vi "Init Prefs.vi"(8 "error in (no error)":errorcluster, 11 "SB App in":refnum<class "SB App.lvclass">) -> (0 "error out":errorcluster, 3 "SB App out":refnum<class "SB App.lvclass">)   [LabVIEW 2020, in "SB App.lvlib" / "SB App.lvclass"]
uses:
  SB App.lvclass
  SB App.lvclass/SB App.ctl
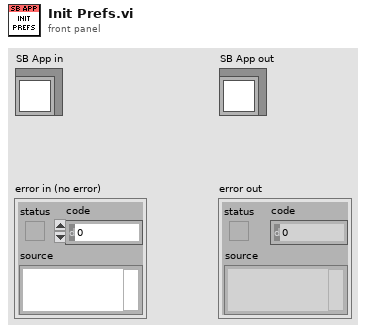
[diagram p1: front panel]
types:
  T1 = enum16{"open", "replace", "create", "open or create", "replace or create", "replace or create with confirmation"}
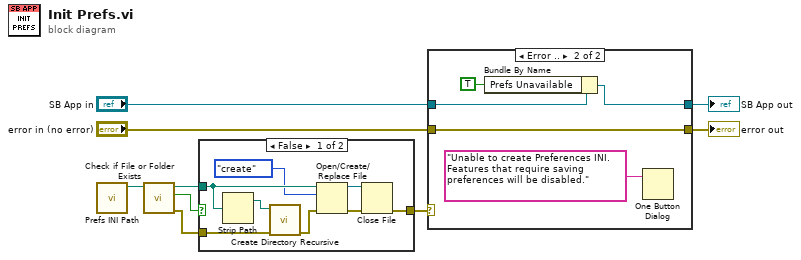
[diagram p0: block diagram]
diagram:
  n1 = call "Prefs INI Path.vi"() -> ("Prefs INI"=w9:path)  [unwired: 11 in]
  n2 = call <vilib>:"Check if File or Folder Exists.vi"("path"=w9) -> ("error out"=w6:errorcluster, "file or folder exists?"=w8:bool, "dup path"=w7:path)  [unwired: 8 in]
  n3 = case shown="False" w8 {
    tunnel: w7 -> [w15 _]
    tunnel: w6 -> [w17 w18]
    tunnel: [w10 w18] -> w5
    frame False {
      n4 = Strip Path(path=w15) -> (stripped path=w16:path)  [unwired: 1 out]
      n5 = call <vilib>:"Create Directory Recursive.vi"("error in (no error)"=w17, "directory"=w16) -> ("error out"=w14:errorcluster)  [unwired: 3 in, 2 out]
      n6 = Open/Create/Replace File(file path (use dialog)=w15, error in=w14, operation (0:open)=T1."create") -> (refnum out=w11:refnum<file>, error out=w12:errorcluster)  [unwired: 3 in, 1 out]
      n7 = Close File(refnum=w11, error in=w12) -> (error out=w10:errorcluster)  [unwired: 1 out]
    }
    frame True {
    }
  }
  n8 = case shown="Error .." w5 {
    tunnel: "error in (no error)" -> [w20 w24]
    tunnel: [w20 w24] -> w3
    tunnel: "SB App in" -> [w19 w23]
    tunnel: [w19 w21] -> w1
    frame No Error {
    }
    frame Error {
      n9 = Bundle By Name(cluster=w23, "Prefs Unavailable"=TRUE) -> (w21:refnum<class "SB App.lvclass">)
      n10 = One Button Dialog(message="Unable to create Preferences INI. Features that require saving preferences will be disabled.") -> ()  [unwired: 1 in, 1 out]
    }
  }
  "error out" <- w3
  "SB App out" <- w1
